vi "test - String Comparison - 01.vi"(8 "error in (no error)":errorcluster, 11 "TestCase in":refnum<class "String Filter Tester.lvclass">) -> (0 "error out":errorcluster, 3 "TestCase out":refnum<class "String Filter Tester.lvclass">)   [LabVIEW 2017, in "String Filter Tester.lvclass"]
uses:
  String Filter Tester.lvclass
  Core/Assert API Components/Filter Configurations/String Filters/String Filters.lvclass
  <vilib>/addons/_JKI Toolkits/VI Tester/TestCase.llb/TestCase.lvclass
  C:/Program Files (x86)/National Instruments/LabVIEW 2017/vi.lib/addons/_JKI Toolkits/VI Tester/TestCase.llb/TestCase.lvclass
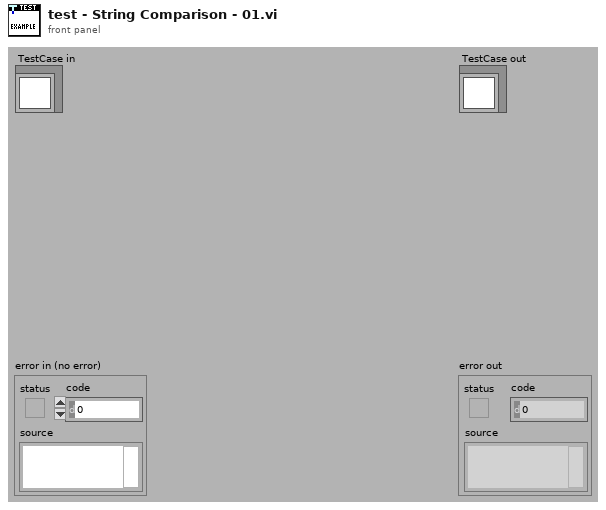
[diagram p1: front panel]
types:
  T1 = enum16{"Contains", "Does Not Contain", "Starts With", "Equals", "Does Not Equal"}
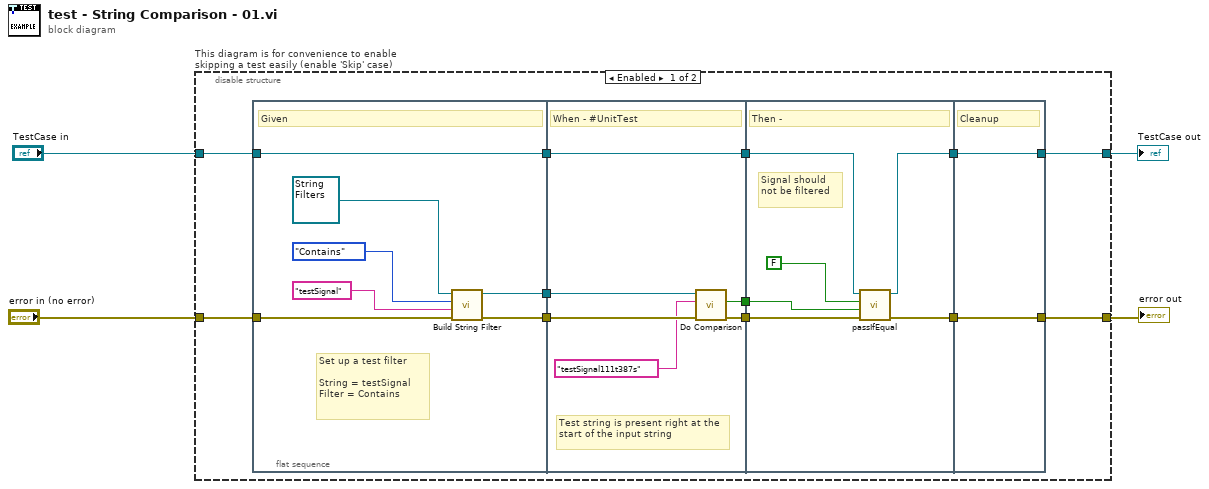
[diagram p0: block diagram]
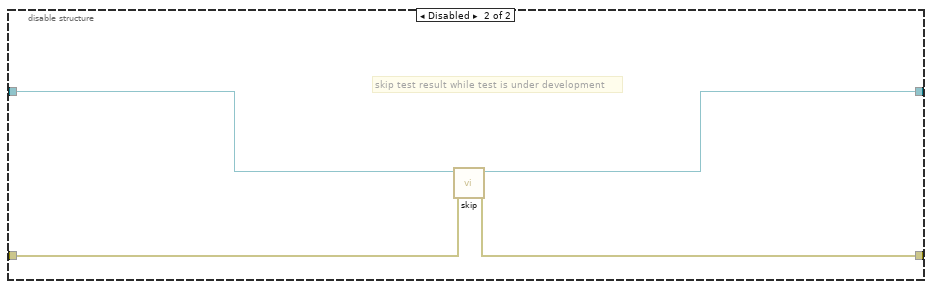
[diagram p2: hidden frame]
diagram:
  n1 = disable-structure "This diagram is for convenience to enable skipping a test easily (enable 'Skip' case)" shown="Enabled" {
    disable-tunnel: "TestCase in" -> [w10 w41]
    disable-tunnel: [w7 w39] -> w1
    disable-tunnel: [w8 w40] -> w3
    disable-tunnel: "error in (no error)" -> [w9 w38]
    frame Enabled {
      n2 = flat-sequence {
        tunnel: w9 -> [w22]
        tunnel: w10 -> [w23]
        tunnel: [w23] -> w16
        tunnel: [w21] -> w15
        tunnel: [w17] -> w6
        tunnel: [w29] -> w14
        tunnel: [w27] -> w13
        tunnel: w16 -> [w29]
        tunnel: w15 -> [w28]
        tunnel: w6 -> [w26]
        tunnel: [w24] -> w5
        tunnel: [w34] -> w12
        tunnel: [w32] -> w11
        tunnel: w14 -> [w35]
        tunnel: w13 -> [w33]
        tunnel: w5 -> [w31]
        tunnel: [w36] -> w8
        tunnel: [w37] -> w7
        tunnel: w12 -> [w37]
        tunnel: w11 -> [w36]
        frame #0 {
          # "Set up a test filter\n\nString = testSignal \nFilter = Contains"
          # "Given"
          n3 = call-dynamic "Build String Filter.vi"("error in (no error)"=w22, "Comparison Value"="testSignal", "Comparison Method"=T1."Contains", "String Filters in"=refnum<class "String Filters.lvclass"> refnum) -> ("error out"=w21:errorcluster, "String Filters out"=w17:refnum<class "String Filters.lvclass">)  [unwired: 6 in]
        }
        frame #1 {
          # "Test string is present right at the start of the input string"
          # "When - #UnitTest"
          n4 = call "Do Comparison.vi"("error in (no error)"=w28, "Compare String"="testSignal111t387s", "String Filters in"=w26) -> ("error out"=w27:errorcluster, "Filtered"=w24:bool)  [unwired: 7 in]
        }
        frame #2 {
          # "Signal should not be filtered"
          # "Then -"
          n5 = call-dynamic "passIfEqual.vi"("error in (no error)"=w33, "y"=w31, "x"=FALSE, "TestCase in"=w35) -> ("error out"=w32:errorcluster, "TestCase out"=w34:refnum<class "String Filter Tester.lvclass">)  [unwired: 6 in]
        }
        frame #3 {
          # "Cleanup"
        }
      }
    }
    frame Disabled {
      # "skip test result while test is under development"
      n6 = call <vilib>:"skip.vi"("error in (no error)"=w38, "TestCase in"=w41) -> ("error out"=w40:errorcluster, "TestCase out"=w39:refnum<class "String Filter Tester.lvclass">)  [unwired: 8 in]
    }
  }
  "error out" <- w3
  "TestCase out" <- w1
